vi "UHR-Fleezers Control (host) -TL FB Corrected Ronen semipassive.vi"(0 "Tab Control":T5(tab)=enum."Trap Control (RF)") -> ()   [LabVIEW 2013] (continued)
                    n948 = Wait (ms)(milliseconds to wait=u32 500) -> ()  [unwired: 1 out]
                  }
                  frame #4 {
                    n949 = call "Write to pump.vi"("string"="start", "VISA resource name"=w1515) -> ()  [unwired: 1 out]
                  }
                }
              }
            }
          }
          frame Enabled {
            n950 = call "hamilton_controller.vi"("Open?"=w1517, "valve"=enum16{"A", "B", "C", "D", "ALL"}."A", "action"=T21."MOVE VALVE") -> ()  [unwired: 8 in, 1 out]
          }
        }
      }
      event "Inject Valve B": Value Change {
        n951 = event-data() -> ()  [unwired: 7 out]
        n952 = disable-structure shown="Enabled" {
          disable-tunnel: "Inject Valve B" -> [w1521 w1541]
          frame Disabled {
            n953 = local read "Pump write delay (ms)"() -> (w1523:dbl)
            n954 = flat-sequence {
              tunnel: w1522 -> [w1536]
              tunnel: w1523 -> [w1532]
              tunnel: w1521 -> [_]
              tunnel: w1523 -> [w1538]
              tunnel: w1522 -> [w1539]
              frame #0 {
                n955 = local read "All Pump Parameters"() -> (w1531:T6)
                n956 = Multiply(x=60.0, y="Flush Center Ch Rate (ul/m)") -> (x*y=w1528:dbl)
                n957 = Unbundle By Name(w1531) -> ("Pump 2"=w1537:T33)
                n958 = call "Set pump parameters.vi"("Pump write delay (ms)"=w1532, "Volume (uL)"="Flush Center Ch Volume (uL)", "Rate (uL/h)"=w1528, "Units"=3.0, "Pump #"=2.0, "Pump Parameters In"=w1537, "VISA resource name"=w1536) -> ("Pump Parameters Out"=w1530:T33)  [unwired: 3 in]
                n959 = Bundle By Name(cluster=w1531, "Pump 2"=w1530) -> (w1529:T6)
                n960 = local write "All Pump Parameters"(w1529) -> ()
                n961 = Add(x="Flush Center Ch Volume (uL)", y="Total Volume\nFlushed (uL)") -> (x+y=w1525:dbl)
                n962 = local write "Total Volume\nFlushed (uL)"(w1525) -> ()
              }
              frame #1 {
                n963 = Wait (ms)(milliseconds to wait=w1538) -> ()  [unwired: 1 out]
              }
              frame #2 {
                n964 = call "Write to pump.vi"("string"="start", "VISA resource name"=w1539) -> ()  [unwired: 1 out]
              }
            }
            n965 = local read "Chemyx Syringe Pump Serial Port"() -> (w1522:refnum<visa-resource-name>)
          }
          frame Enabled {
            n966 = call "hamilton_controller.vi"("Open?"=w1541, "valve"=enum16{"A", "B", "C", "D", "ALL"}."B", "action"=T21."MOVE VALVE") -> ()  [unwired: 8 in, 1 out]
          }
        }
      }
      event "Inject Bottom": Value Change {
        n967 = event-data() -> ()  [unwired: 7 out]
        n968 = call "hamilton_controller.vi"("Open?"="Inject Bottom", "valve"=enum16{"A", "B", "C", "D", "ALL"}."C", "action"=T21."MOVE VALVE") -> ()  [unwired: 8 in, 1 out]
      }
      event "Shunt:": Value Change {
        n969 = event-data() -> ()  [unwired: 7 out]
        n970 = call "hamilton_controller.vi"("Open?"="Shunt:", "valve"=enum16{"A", "B", "C", "D", "ALL"}."D", "action"=T21."MOVE VALVE") -> ()  [unwired: 8 in, 1 out]
      }
      event "Flip Green Filter": Value Change {
        n971 = event-data() -> ()  [unwired: 7 out]
        n972 = local write "Flip Green Filter"("Flip Green Filter") -> ()
        n973 = flat-sequence {
          tunnel: w1557 -> [w1562]
          tunnel: w1556 -> [w1561]
          tunnel: [w1559] -> w1554
          tunnel: [w1558] -> w1553
          tunnel: [w1564] -> w1552
          tunnel: w1554 -> [w1564]
          tunnel: [w1563] -> w1551
          tunnel: w1553 -> [w1563]
          tunnel: w1552 -> [w1568]
          tunnel: w1551 -> [w1567]
          tunnel: [w1566] -> w1555
          frame #0 {
            n974 = xnode "Read/Write Control"("FPGA VI Reference In"=w1562, "error in"=w1561, "Green Filter Flipper"=TRUE) -> ("FPGA VI Reference Out"=w1559:T20, "error out"=w1558:errorcluster)
          }
          frame #1 {
            n975 = Wait (ms)(milliseconds to wait=u32 100) -> ()  [unwired: 1 out]
          }
          frame #2 {
            n976 = xnode "Read/Write Control"("FPGA VI Reference In"=w1568, "error in"=w1567, "Green Filter Flipper"=FALSE) -> ("error out"=w1566:errorcluster)  [unwired: 1 out]
          }
        }
      }
      event "Pump 1 contents", "Pump 3 contents": Value Change {
        n977 = event-data() -> ()  [unwired: 7 out]
        n978 = local read "Pump 1 contents"() -> (→"Pump 1 cont disp":string)
        n979 = local read "Pump 3 contents"() -> (→"Pump 3 cont disp":string)
      }
      event "Reset Trap Pos. FB": Value Change {
        n980 = event-data() -> ()  [unwired: 7 out]
        n981 = xnode "Read/Write Control"("FPGA VI Reference In"=w1574, "error in"=w1573, "Trap Pos. FB Reset"="Reset Trap Pos. FB") -> ()  [unwired: 2 out]
      }
      event "Trap Pos. FB ON": Value Change {
        n982 = event-data() -> ()  [unwired: 7 out]
        n983 = xnode "Read/Write Control"("FPGA VI Reference In"=w1589, "error in"=w1588) -> ("FPGA VI Reference Out"=w1586:T20, "BD1 Frequency Out 1"=w1583:u64)  [unwired: 1 out]
        n984 = To Double Precision Float(number=w1583) -> (double precision float=w1582:dbl)
        n985 = Multiply(x=49125000.0, y=6.0) -> (x*y=w1581:dbl)
        n986 = Multiply(x=w1582, y=w1581) -> (x*y=w1579:dbl)
        n987 = Scale By Power Of 2(n=-48, x=w1579) -> (x*2^n=w1578:dbl)
        n988 = Divide(x=w1578, y=1000000.0) -> (x/y=w1575:dbl)
        n989 = flat-sequence {
          tunnel: [w1592] -> w1587
          tunnel: w1586 -> [w1593]
          tunnel: w1583 -> [w1591]
          tunnel: "Trap Pos. FB ON" -> [w1590]
          tunnel: "Trap Pos. FB ON" -> [w1599]
          tunnel: w1587 -> [w1598]
          tunnel: "Trap Pos. FB ON" -> [w1601]
          tunnel: w1575 -> [w1600]
          frame #0 {
            n990 = case shown="False" w1590 {
              tunnel: w1593 -> [w1596 w1597]
              tunnel: [w1595 w1597] -> w1592
              tunnel: w1591 -> [w1594 _]
              frame False {
                n991 = xnode "Read/Write Control"("FPGA VI Reference In"=w1596, "BD 1 Frequency 1"=w1594) -> ("FPGA VI Reference Out"=w1595:T20)  [unwired: 1 in, 1 out]
              }
              frame True {
              }
            }
          }
          frame #1 {
            n992 = xnode "Read/Write Control"("FPGA VI Reference In"=w1598, "Force feedback"=w1599) -> ()  [unwired: 1 in, 2 out]
          }
          frame #2 {
            n993 = case shown="False" w1601 {
              tunnel: w1600 -> [w1603 _]
              frame False {
                n994 = Subtract(x=90.0, y=w1603) -> (x-y=w1602:dbl)
                n995 = property on="Trap Delta (MHz)" class="DigNum (strict)"("Val(Sgnl)"=w1602) -> ()  [unwired: 2 in, 2 out]
              }
              frame True {
              }
            }
          }
        }
      }
      event "Diff. FB.", "Trap Pos. FB Gains", "Trap Pos. FB Mult Factor", "Trap Pos. FB Offset Factor", "Trap Pos FB Negate Action", "Trap Pos FB Monitor\nT1 or T2", "Negate Diff?": Value Change {
        n996 = event-data() -> ()  [unwired: 7 out]
        n997 = xnode "Read/Write Control"("FPGA VI Reference In"=w1615, "error in"=w1614, "Trap Pos. FB Range"="Trap Pos. FB Range", "Trap Pos. FB Gains"="Trap Pos. FB Gains", "Trap Pos. FB Mult Factor"="Trap Pos. FB Mult Factor", "Trap Pos. FB Offset Factor"="Trap Pos. FB Offset Factor", "Trap Pos FB Negate Action"="Trap Pos FB Negate Action", "Trap Pos FB Monitor T1 or T2"="Trap Pos FB Monitor\nT1 or T2", "AI1 X Scale"="Trap Pos. AI1 X Pre-scale", "Negate Diff?"="Negate Diff?", "Diff FB Measurement?"="Diff. FB.") -> ()  [unwired: 2 out]
      }
      event "Trap Pos FB SP": Value Change {
        n998 = event-data() -> ()  [unwired: 7 out]
        n999 = xnode "Read/Write Control"("FPGA VI Reference In"=w1618, "error in"=w1617, "Trap Pos. FB SP"="Trap Pos FB SP") -> ()  [unwired: 2 out]
      }
      event "Set SP to Reading": Value Change {
        n1000 = event-data() -> ()  [unwired: 7 out]
        n1001 = local read "Trap Pos FB Monitor\nT1 or T2"() -> (w1626:bool)
        n1002 = local read "Trap X AI1 (DMA)"() -> (w1629:T13)
        n1003 = local read "Trap X (AI1)"() -> (w1632:T1)
        n1004 = Unbundle By Name(w1632) -> ("Trap 1"=w1631:fxp<+/-,16,1>, "Trap 2"=w1630:fxp<+/-,16,1>)
        n1005 = Unbundle By Name(w1629) -> ("Set 1"=w1628:fxp<+/-,16,1>, "Set 2"=w1627:fxp<+/-,16,1>)
        n1006 = Select(t=w1631, s=w1626, f=w1630) -> (s? t:f=w1625:fxp<+/-,16,1>)
        n1007 = Select(t=w1628, s=w1626, f=w1627) -> (s? t:f=w1624:fxp<+/-,16,1>)
        n1008 = Not(x="Set SP Using...") -> (.not. x?=w1619:bool)
        n1009 = Select(t=w1625, s=w1619, f=w1624) -> (s? t:f=w1620:fxp<+/-,16,1>)
        n1010 = xnode "Read/Write Control"("FPGA VI Reference In"=w1622, "error in"=w1621, "Trap Pos. FB SP"=w1620) -> ()  [unwired: 2 out]
        n1011 = local write "Trap Pos FB SP"(w1620) -> ()
      }
      event "Trap Pos. FB Out Scale 2^n": Value Change {
        n1012 = event-data() -> ()  [unwired: 7 out]
        n1013 = Scale By Power Of 2(n="Trap Pos. FB Out Scale 2^n", x=ext 1.0) -> (x*2^n=w1634:ext)
        n1014 = property on="Trap Pos. FB Mult Factor" class="DigNum (strict)"("Val(Sgnl)"=w1634) -> ()  [unwired: 2 in, 2 out]
      }
      event "Trap Pos FB Int Count": Value Change {
        n1015 = event-data() -> ()  [unwired: 7 out]
        n1016 = xnode "Read/Write Control"("FPGA VI Reference In"=w1639, "error in"=w1638, "Trap Pos FB Int Count"="Trap Pos FB Int Count") -> ()  [unwired: 2 out]
      }
      event "Target Force (pN)", "Setpoint offset\nCorrection values": Value Change {
        n1017 = event-data() -> ()  [unwired: 7 out]
        n1018 = local read "B factor"() -> (w1672:dbl)
        n1019 = To Fixed-Point(number=w1672) -> (fixed-point=w1671:fxp<+/-,16,16>)  [unwired: 1 in]
        n1020 = xnode "Read/Write Control"("FPGA VI Reference In"=w1673, "B factor"=w1671) -> ("BD1 Frequency Out 1"=w1662:u64)  [unwired: 1 in, 2 out]
        n1021 = local read "BD 1 Frequency 2 (MHz)"() -> (w1661:dbl)
        n1022 = local read "Target Force (pN)"() -> (w1647:dbl)
        n1023 = To Double Precision Float(number=w1662) -> (double precision float=w1668:dbl)
        n1024 = Multiply(x=49125000.0, y=6.0) -> (x*y=w1667:dbl)
        n1025 = Multiply(x=w1668, y=w1667) -> (x*y=w1665:dbl)
        n1026 = Scale By Power Of 2(n=-48, x=w1665) -> (x*2^n=w1664:dbl)
        n1027 = Divide(x=w1664, y=1000000.0) -> (x/y=w1660:dbl)
        n1028 = Subtract(x=w1661, y=w1660) -> (x-y=w1659:dbl)
        n1029 = local read "T1 kappa_x (pN/nm)"() -> (w1648:dbl)
        n1030 = local read "T1 alpha_x (nm/V)"() -> (w1649:dbl)
        n1031 = local read "Negate offset difference"() -> (w1650:bool)
        n1032 = local read "Offset file step size"() -> (w1658:dbl)
        n1033 = Multiply(x=w1647, y=2.0) -> (x*y=w1645:dbl)
        n1034 = local read "Setpoint offset\nCorrection values"() -> (w1655:dbl[])
        n1035 = Divide(x=w1659, y=w1658) -> (x/y=w1657:dbl)
        n1036 = Select(t=-1, s=w1650, f=1) -> (s? t:f=w1651:i32)
        n1037 = To Long Integer(number=w1657) -> (32bit integer=w1656:i32)
        n1038 = Multiply(x=w1649, y=w1648) -> (x*y=w1644:dbl)
        n1039 = Divide(x=w1645, y=w1644) -> (x/y=w1643:dbl)
        n1040 = Index Array(array=w1655, index=w1656) -> (element=w1654:dbl)
        n1041 = Multiply(x=w1651, y=w1654) -> (x*y=w1642:dbl)
        n1042 = Add(x=w1643, y=w1642) -> (x+y=w1641:dbl)
        n1043 = To Fixed-Point(number=w1641) -> (fixed-point=w1640:fxp<+/-,16,1>)  [unwired: 1 in]
        n1044 = property on="Trap Pos FB SP" class="DigNum (strict)"("Val(Sgnl)"=w1640) -> ()  [unwired: 2 in, 2 out]
      }
      event "Read setpoint correction\nfile": Value Change {
        n1045 = event-data() -> ()  [unwired: 7 out]
        n1046 = local write "Read setpoint correction\nfile"(FALSE) -> ()
        n1047 = Open/Create/Replace File(file path (use dialog)="Setpoint correction\noffset file", operation (0:open)=T24."open", access (0:read/write)=enum16{"read/write", "read-only", "write-only"}."read-only") -> (refnum out=w1698:refnum<file>)  [unwired: 1 in, 4 out]
        n1048 = Deny Access(7:w1698) -> (3:w1696:refnum<file>)  [unwired: 1 in, 2 out]
        n1049 = Read from Binary File(5:0.0, 9:T30."big-endian, network order" ("byte order (0:big-endian, network order)"), 10:-1 ("count (1)"), 11:w1696) -> (2:w1689:dbl[], 3:w1695:refnum<file>)  [unwired: 1 in, 3 out]
        n1050 = Close File(refnum=w1695) -> ()  [unwired: 1 in, 2 out]
        n1051 = Index Array(array=w1689, index=0) -> (element=w1685:dbl)
        n1052 = local write "Offset file step size"(w1685) -> ()
        n1053 = Array Subset(array=w1689, index=3) -> (w1688:dbl[])  [unwired: 1 in]
        n1054 = local read "T1 kappa_x (pN/nm)"() -> (w1683:dbl)
        n1055 = local read "T1 alpha_x (nm/V)"() -> (w1684:dbl)
        n1056 = local read "T2 alpha_x (nm/V)"() -> (w1682:dbl)
        n1057 = local read "T2 kappa_x (pN/nm)"() -> (w1681:dbl)
        n1058 = Decimate 1D Array(w1688) -> (w1676:dbl[], w1677:dbl[])  [unwired: 1 out]
        n1059 = local read "Offset Values"() -> (w1687:T14)
        n1060 = Multiply(x=w1684, y=w1683) -> (x*y=w1679:dbl)
        n1061 = Multiply(x=w1682, y=w1681) -> (x*y=w1680:dbl)
        n1062 = Bundle By Name(cluster=w1687, "Trap 1X offset"=w1676, "Trap 2X offset"=w1677) -> (w1686:T14)
        n1063 = Divide(x=w1680, y=w1679) -> (x/y=w1678:dbl)
        n1064 = property on="B factor" class="DigNum (strict)"("Val(Sgnl)"=w1678) -> ()  [unwired: 2 in, 2 out]
        n1065 = Multiply(x=w1677, y=w1678) -> (x*y=w1675:dbl[])
        n1066 = local write "Offset Values"(w1686) -> ()
        n1067 = Subtract(x=w1676, y=w1675) -> (x-y=w1674:dbl[])
        n1068 = property on="Setpoint offset\nCorrection values" class="Arr (strict)"("Val(Sgnl)"=w1674) -> ()  [unwired: 2 in, 2 out]
      }
      event "MCL Tracking": Value Change {
        n1069 = event-data() -> ()  [unwired: 7 out]
        n1070 = case shown="True" "MCL Tracking" {
          frame False {
            n1071 = local read "Current MCL (V)"() -> (w1703:dbl)
            n1072 = local write "AO2"(w1703) -> ()
          }
          frame True {
            n1073 = local read "BD 1 Frequency 1 (MHz)"() -> (→"Zero T1 position":dbl)
            n1074 = local read "AO2"() -> (→"Zero MCL x position":dbl)
          }
        }
      }
    }
    "error out 2" <- w754
    n1075 = node-c288() -> ()  [unwired: 1 in, 1 out]
  }
  n1076 = timed-loop "Run Scripts, including: stage motion" {
    timing: w89 -> [_]
    timing-out: [_] -> w88
    tunnel: w44 -> [_]
    stop <- w1707 stop-if-true
    n1077 = node-c288() -> ()  [unwired: 1 in, 1 out]
    n1078 = event shown="[2] \"Cal/Data Acq. Spot\": Value Change" {
      selector: _ -> [_ _ _ _ _ _ _ _ _ _ _ _]
      dyn-events: _ -> [_ _ _ _ _ _ _ _ _ _ _ _]
      timeout: 50 -> [_ _ _ _ _ _ _ _ _ _ _ _]
      tunnel: ["Move Cap. 1 (DNA Top)" _ "Cal/Data Acq. Spot" "Dump Beads" "Dip for Protein" _ "Got ADig bead" "Got DNA bead" "Take Stepping Data" _ "Take Detection Laser\nImage" _] -> _
      tunnel: [_ _ _ _ _ _ _ _ _ _ _ w1915] -> w1707
      event "Move Cap. 1 (DNA Top)": Value Change {
        n1079 = event-data() -> ()  [unwired: 1 in, 5 out]
        n1080 = local write "Move Cap. 1 (DNA Top)"(FALSE ("Move Cap. 1 (DNA Right)")) -> ()
        n1081 = flat-sequence {
          tunnel: "Cap 1 Samp Flow ON" -> [w1713]
          frame #0 {
            n1082 = local write "Stage Moving"(FALSE ("Stage Moving")) -> ()
            n1083 = case "stop flow" shown="True" w1713 {
              frame False {
              }
              frame True {
                n1084 = call "hamilton_controller.vi"("Open?"=FALSE, "valve"=enum16{"A", "B", "C", "D", "ALL"}."C", "action"=T21."MOVE VALVE") -> ()  [unwired: 8 in, 1 out]
              }
            }
            n1085 = case shown="True" TRUE {
              tunnel: "Cap 1 T ON" -> [w1722 w1723]
              frame False {
                n1086 = property on="Trap 1 (ON/OFF)" class="Bool (strict)"("Val(Sgnl)"=w1722) -> ()  [unwired: 2 in, 2 out]
              }
              frame True {
                n1087 = property on="Trap 2 (ON/OFF)" class="Bool (strict)"("Val(Sgnl)"=w1723) -> ()  [unwired: 2 in, 2 out]
              }
            }
            n1088 = call <vilib>:"Beep.vi"() -> ()  [unwired: 3 in, 9 out]
            n1089 = case shown="True" "Cap 1 Flow ON" {
              frame False {
              }
              frame True {
                n1090 = property on="Main:" class="Bool (strict)"("Val(Sgnl)"=TRUE ("Value (Signaling)")) -> ()  [unwired: 2 in, 2 out]
              }
            }
          }
        }
      }
      event Timeout {
        n1091 = event-data() -> ()  [unwired: 1 in, 2 out]
      }
      event "Cal/Data Acq. Spot": Value Change {
        # "wait for calibration file\nto be written"
        # "signal save cal true\nthis tells the data \nacquisition loop to\nstart sending the data\nto a calibration file"
        # "separate traps to\nthe desired trap delta"
        # "move stage to data acquisition spot"
        # "CHANGE FISH FOR TETHER BACK\nTO TRUE VALUE HERE."
        n1092 = event-data() -> ()  [unwired: 1 in, 5 out]
        n1093 = local write "Cal/Data Acq. Spot"(FALSE ("Cal/Data Acq. Spot")) -> ()
        n1094 = flat-sequence {
          tunnel: ["Cal @ (MHz)"] -> w1724
          tunnel: w1724 -> [w1734]
          tunnel: w1724 -> [w1755]
          frame #0 {
            n1095 = property on="Trap Delta (MHz)" class="DigNum (strict)"("Val(Sgnl)"="Cal @ (MHz)") -> ()  [unwired: 2 in, 2 out]
            n1096 = call <vilib>:"Beep.vi"() -> ()  [unwired: 3 in, 9 out]
          }
          frame #1 {
            n1097 = Wait (ms)(milliseconds to wait=u32 100) -> ()  [unwired: 1 out]
          }
          frame #2 {
            n1098 = property on="Save Calibration" class="Bool (strict)"("Val(Sgnl)"=TRUE ("Value (Signaling)")) -> ()  [unwired: 2 in, 2 out]
          }
          frame #3 {
            n1099 = Wait (ms)(milliseconds to wait=u32 4000) -> ()  [unwired: 1 out]
          }
          frame #4 {
            n1100 = while {
              stop <- w1731 stop-if-true
              n1101 = local read "Saving..."() -> (w1732:bool)
              n1102 = Wait (ms)(milliseconds to wait=u32 100) -> ()  [unwired: 1 out]
              n1103 = Not(x=w1732) -> (.not. x?=w1731:bool)
            }
          }
          frame #5 {
            n1104 = case shown="True" "W/ Offset 1" {
              tunnel: w1734 -> [_ w1736]
              frame False {
              }
              frame True {
                n1105 = stacked-sequence {
                  tunnel: w1736 -> [_ _ _ _ _ _ _ w1753]
                  frame #0 {
                    n1106 = Replace Array Subset(array=u32[] [0] ("Index Values"), new element="Offset 1 Set", index=0) -> (w1737:u32[])
                    n1107 = property on="Saved AOD Raster Scan Parameter Sets" class="Arr (strict)"("Index Values"=w1737) -> ()  [unwired: 2 in, 2 out]
                    n1108 = property on="Trap Delta (MHz)" class="DigNum (strict)"("Val(Sgnl)"="Offset 1 Start (MHz)") -> ()  [unwired: 2 in, 2 out]
                  }
                  frame #1 {
                    n1109 = Wait (ms)(milliseconds to wait=u32 200) -> ()  [unwired: 1 out]
                  }
                  frame #2 {
                    n1110 = property on="Load parameters" class="Bool (strict)"("Val(Sgnl)"=TRUE ("Value (Signaling)")) -> ()  [unwired: 2 in, 2 out]
                  }
                  frame #3 {
                    n1111 = Wait (ms)(milliseconds to wait=u32 200) -> ()  [unwired: 1 out]
                  }
                  frame #4 {
                    n1112 = property on="Trap Raster Scan" class="Bool (strict)"("Val(Sgnl)"=TRUE ("Value (Signaling)")) -> ()  [unwired: 2 in, 2 out]
                  }
                  frame #5 {
                    n1113 = Wait (ms)(milliseconds to wait=u32 2000) -> ()  [unwired: 1 out]
                  }
                  frame #6 {
                    n1114 = while {
                      stop <- w1750 stop-if-true
                      n1115 = local read "Raster Scanning..."() -> (w1752:bool)
                      n1116 = local read "Saving..."() -> (w1748:bool)
                      n1117 = Wait (ms)(milliseconds to wait=u32 100) -> ()  [unwired: 1 out]
                      n1118 = Not(x=w1748) -> (.not. x?=w1747:bool)
                      n1119 = Not(x=w1752) -> (.not. x?=w1749:bool)
                      n1120 = And(x=w1749, y=w1747) -> (x .and. y?=w1750:bool)
                    }
                  }
                  frame #7 {
                    n1121 = property on="Trap Delta (MHz)" class="DigNum (strict)"("Val(Sgnl)"=w1753) -> ()  [unwired: 2 in, 2 out]
                  }
                }
              }
            }
          }
          frame #6 {
            n1122 = local read "Save ave N"() -> (w1754:dbl)
            n1123 = case shown="True" "W/ Offset 2" {
              tunnel: w1755 -> [_ w1761]
              tunnel: w1754 -> [_ w1760]
              frame False {
                n1124 = Multiply(x="Cal read wait (s)", y=u32 1000 ("milliseconds to wait")) -> (x*y=w1758:u32)
                n1125 = Wait (ms)(milliseconds to wait=w1758) -> ()  [unwired: 1 out]
              }
              frame True {
                n1126 = stacked-sequence {
                  tunnel: w1761 -> [_ _ _ _ _ _ _ _ _ w1782 _ _]
                  tunnel: w1760 -> [_ _ _ _ _ _ _ _ _ w1780 _ _]
                  frame #0 {
                    n1127 = property on="Save ave N" class="DigNum (strict)"("Val(Sgnl)"=1.0 ("Value (Signaling)")) -> ()  [unwired: 2 in, 2 out]
                  }
                  frame #1 {
                    n1128 = Wait (ms)(milliseconds to wait=u32 500) -> ()  [unwired: 1 out]
                  }
                  frame #2 {
                    n1129 = property on="Trap Delta (MHz)" class="DigNum (strict)"("Val(Sgnl)"="Offset 2 Start (MHz)") -> ()  [unwired: 2 in, 2 out]
                    n1130 = Replace Array Subset(array=u32[] [0] ("Index Values"), new element="Offset 2 Set", index=0) -> (w1766:u32[])
                    n1131 = property on="Saved AOD Raster Scan Parameter Sets" class="Arr (strict)"("Index Values"=w1766) -> ()  [unwired: 2 in, 2 out]
                  }
                  frame #3 {
                    n1132 = Wait (ms)(milliseconds to wait=u32 500) -> ()  [unwired: 1 out]
                  }
                  frame #4 {
                    n1133 = property on="Load parameters" class="Bool (strict)"("Val(Sgnl)"=TRUE ("Value (Signaling)")) -> ()  [unwired: 2 in, 2 out]
                  }
                  frame #5 {
                    n1134 = Wait (ms)(milliseconds to wait=u32 500) -> ()  [unwired: 1 out]
                  }
                  frame #6 {
                    n1135 = property on="Trap Raster Scan" class="Bool (strict)"("Val(Sgnl)"=TRUE ("Value (Signaling)")) -> ()  [unwired: 2 in, 2 out]
                  }
                  frame #7 {
                    n1136 = Wait (ms)(milliseconds to wait=u32 2000) -> ()  [unwired: 1 out]
                  }
                  frame #8 {
                    n1137 = while {
                      stop <- w1775 stop-if-true
                      n1138 = local read "Raster Scanning..."() -> (w1778:bool)
                      n1139 = local read "Saving..."() -> (w1776:bool)
                      n1140 = Wait (ms)(milliseconds to wait=u32 100) -> ()  [unwired: 1 out]
                      n1141 = Not(x=w1776) -> (.not. x?=w1774:bool)
                      n1142 = Not(x=w1778) -> (.not. x?=w1777:bool)
                      n1143 = And(x=w1777, y=w1774) -> (x .and. y?=w1775:bool)
                    }
                  }
                  frame #9 {
                    n1144 = property on="Trap Delta (MHz)" class="DigNum (strict)"("Val(Sgnl)"=w1782) -> ()  [unwired: 2 in, 2 out]
                    n1145 = property on="Saved AOD Raster Scan Parameter Sets" class="Arr (strict)"("Index Values"=u32[] [0]) -> ()  [unwired: 2 in, 2 out]
                    n1146 = property on="Save ave N" class="DigNum (strict)"("Val(Sgnl)"=w1780) -> ()  [unwired: 2 in, 2 out]
                  }
                  frame #10 {
                    n1147 = Wait (ms)(milliseconds to wait=u32 500) -> ()  [unwired: 1 out]
                  }
                  frame #11 {
                    n1148 = property on="Load parameters" class="Bool (strict)"("Val(Sgnl)"=TRUE ("Value (Signaling)")) -> ()  [unwired: 2 in, 2 out]
                  }
                }
              }
            }
          }
          frame #7 {
            n1149 = property on="Read Cal" class="Bool (strict)"("Val(Sgnl)"=TRUE ("Value (Signaling)")) -> ()  [unwired: 2 in, 2 out]
          }
          frame #8 {
            n1150 = Wait (ms)(milliseconds to wait=u32 500) -> ()  [unwired: 1 out]
          }
          frame #9 {
            n1151 = property on="Fish for Tether" class="Bool (strict)"("Val(Sgnl)"=FALSE ("Value (Signaling)")) -> ()  [unwired: 2 in, 2 out]
          }
        }
      }
      event "Dump Beads": Value Change {
        # "SCRIPT TO REMOVE BOTH BEADS FROM THE TRAPS. TURNS ON LIGHT WHICH INDICATES THAT STAGE IS MOVING. THEN STOPS SAVING DATA. \nSETS Sample Channel Flow TO TRUE. STOPS INTERLACING GREEN FLUORESCENCE. TURNS OFF Tether INDICATOR BECAUSE WE ARE THROWING IT\nAWAY. SHUTS OFF TRAP POSITION FEEDBACK."
        n1152 = event-data() -> ()  [unwired: 1 in, 5 out]
        n1153 = flat-sequence {
          frame #0 {
            w1789 = FALSE ("Fl. Triggered...")
            w1790 = TRUE ("Stage Moving")
            n1154 = local read "Saving..."() -> (w1791:bool)
            n1155 = local write "Fl. Triggered..."(w1789) -> ()
            n1156 = local write "Stage Moving"(w1790) -> ()
            n1157 = local write "Tether"(w1789) -> ()
            n1158 = property on="Green Laser ON/Interlacing" class="Bool (strict)"("Val(Sgnl)"=w1789) -> ()  [unwired: 2 in, 2 out]
            n1159 = property on="Trap Pos. FB ON" class="Bool (strict)"("Val(Sgnl)"=w1789) -> ()  [unwired: 2 in, 2 out]
            n1160 = property on="Inject Bottom" class="Bool (strict)"("Val(Sgnl)"=w1790) -> ()  [unwired: 2 in, 2 out]
            n1161 = local write "Stop Saving"(w1791) -> ()
          }
          frame #1 {
            w1792 = FALSE ("Value (Signaling)")
            # "TURNS TRAPS OFF SO THAT\nBEADS REMAIN AT DUMP \nBEADS POSITION"
            n1162 = property on="Trap 1 (ON/OFF)" class="Bool (strict)"("Val(Sgnl)"=w1792) -> ()  [unwired: 2 in, 2 out]
            n1163 = property on="Trap 2 (ON/OFF)" class="Bool (strict)"("Val(Sgnl)"=w1792) -> ()  [unwired: 2 in, 2 out]
            n1164 = call <vilib>:"Beep.vi"() -> ()  [unwired: 3 in, 9 out]
          }
          frame #2 {
            n1165 = property on="Goto Bottom (F7)" class="Bool (strict)"("Val(Sgnl)"=TRUE ("Value (Signaling)")) -> ()  [unwired: 2 in, 2 out]
          }
          frame #3 {
            n1166 = Wait (ms)(milliseconds to wait=u32 8000) -> ()  [unwired: 1 out]
          }
          frame #4 {
            n1167 = property on="Trap Delta (MHz)" class="DigNum (strict)"("Val(Sgnl)"=20.0 ("Value (Signaling)")) -> ()  [unwired: 2 in, 2 out]
          }
          frame #5 {
            n1168 = property on="Trap 2 (ON/OFF)" class="Bool (strict)"("Val(Sgnl)"=TRUE ("Value (Signaling)")) -> ()  [unwired: 2 in, 2 out]
          }
          frame #6 {
            n1169 = property on="Inject Bottom" class="Bool (strict)"("Val(Sgnl)"=FALSE ("Value (Signaling)")) -> ()  [unwired: 2 in, 2 out]
          }
        }
      }
      event "Dip for Protein": Value Change {
        n1170 = event-data() -> ()  [unwired: 1 in, 5 out]
        n1171 = flat-sequence {
          frame #0 {
            n1172 = case shown="True" "Move Trap Before?" {
              frame False {
              }
              frame True {
                n1173 = property on="Trap Delta (MHz)" class="DigNum (strict)"("Val(Sgnl)"="Dip Trap Delta 1 (MHz)") -> ()  [unwired: 2 in, 2 out]
              }
            }
          }
          frame #1 {
            n1174 = Multiply(x="Duration (s)", y=1000.0) -> (x*y=w1801:dbl)
            n1175 = Wait (ms)(milliseconds to wait=w1801) -> ()  [unwired: 1 out]
          }
          frame #2 {
            n1176 = case shown="True" "Move Trap After?" {
              frame False {
              }
              frame True {
                n1177 = property on="Trap Delta (MHz)" class="DigNum (strict)"("Val(Sgnl)"="Dip Trap Delta 2 (MHz)") -> ()  [unwired: 2 in, 2 out]
              }
            }
          }
          frame #3 {
            n1178 = case shown="True" "Green ON After?" {
              frame False {
              }
              frame True {
                n1179 = property on="Green Laser ON/Interlacing" class="Bool (strict)"("Val(Sgnl)"=TRUE ("Value (Signaling)")) -> ()  [unwired: 2 in, 2 out]
              }
            }
          }
          frame #4 {
            n1180 = Wait (ms)(milliseconds to wait=u32 500) -> ()  [unwired: 1 out]
          }
          frame #5 {
            n1181 = case shown="True" "Save Data After?" {
              frame False {
              }
              frame True {
                n1182 = property on="Start Saving" class="Bool (strict)"("Val(Sgnl)"=TRUE ("Value (Signaling)")) -> ()  [unwired: 2 in, 2 out]
              }
            }
          }
        }
      }
      event "Profile": Value Change {
        n1183 = event-data() -> ()  [unwired: 1 in, 5 out]
        n1184 = flat-sequence {
          frame #0 {
            w1811 = 0.0 ("element")
            n1185 = Build Array(w1811, "Y change (mm)", w1811) -> ()  [unwired: 1 out]
          }
          frame #1 {
            # "stop saving"
            n1186 = local write "Stop Saving"(TRUE ("Stop Saving")) -> ()
            n1187 = local write "Stage Moving"(FALSE ("Stage Moving")) -> ()
          }
        }
      }
      event "Got ADig bead": Value Change {
        n1188 = event-data() -> ()  [unwired: 1 in, 5 out]
        n1189 = property on="Move Cap. 1 (DNA Top)" class="Bool (strict)"("Val(Sgnl)"=TRUE ("Value (Signaling)")) -> ()  [unwired: 2 in, 2 out]
        n1190 = property on="Inject Top:" class="Bool (strict)"("Val(Sgnl)"=FALSE ("Value (Signaling)")) -> ()  [unwired: 2 in, 2 out]
      }
      event "Got DNA bead": Value Change {
        n1191 = event-data() -> ()  [unwired: 1 in, 5 out]
        n1192 = property on="Cal/Data Acq. Spot" class="Bool (strict)"("Val(Sgnl)"=TRUE ("Value (Signaling)")) -> ()  [unwired: 2 in, 2 out]
        n1193 = property on="Main:" class="Bool (strict)"("Val(Sgnl)"=FALSE ("Value (Signaling)")) -> ()  [unwired: 2 in, 2 out]
      }
      event "Take Stepping Data": Value Change {
        n1194 = event-data() -> ()  [unwired: 1 in, 5 out]
        n1195 = local read "Save ave N"() -> (w1829:dbl)
        n1196 = flat-sequence {
          tunnel: w1829 -> [w1831]
          tunnel: [w1831] -> w1824
          tunnel: [w1833] -> w1825
          tunnel: w1824 -> [w1833]
          tunnel: [w1835] -> w1826
          tunnel: w1825 -> [w1835]
          tunnel: [w1838] -> w1827
          tunnel: w1826 -> [w1838]
          tunnel: [w1840] -> w1828
          tunnel: w1827 -> [w1840]
          tunnel: [w1842] -> w1822
          tunnel: w1828 -> [w1842]
          tunnel: w1822 -> [w1845]
          tunnel: [w1845] -> w1821
          tunnel: w1821 -> [w1846]
          tunnel: [w1846] -> w1823
          tunnel: w1823 -> [w1852]
          frame #0 {
            n1197 = property on="Save ave N" class="DigNum (strict)"("Val(Sgnl)"="Save ave factor") -> ()  [unwired: 2 in, 2 out]
          }
          frame #1 {
            n1198 = Wait (ms)(milliseconds to wait=u32 100) -> ()  [unwired: 1 out]
          }
          frame #2 {
            n1199 = local read "Offset 2 Start (MHz)"() -> (w1837:dbl)
            n1200 = property on="Saved AOD Raster Scan Parameter Sets" class="Arr (strict)"("Index Values"=u32[] [2]) -> ()  [unwired: 2 in, 2 out]
            n1201 = property on="Trap Delta (MHz)" class="DigNum (strict)"("Val(Sgnl)"=w1837) -> ()  [unwired: 2 in, 2 out]
          }
          frame #3 {
            n1202 = property on="Load parameters" class="Bool (strict)"("Val(Sgnl)"=TRUE ("Value (Signaling)")) -> ()  [unwired: 2 in, 2 out]
          }
          frame #4 {
            n1203 = Wait (ms)(milliseconds to wait=u32 100) -> ()  [unwired: 1 out]
          }
          frame #5 {
            n1204 = property on="Trap Raster Scan" class="Bool (strict)"("Val(Sgnl)"=TRUE ("Value (Signaling)")) -> ()  [unwired: 2 in, 2 out]
          }
          frame #6 {
            n1205 = Wait (ms)(milliseconds to wait=u32 1000) -> ()  [unwired: 1 out]
          }
          frame #7 {
            n1206 = while {
              stop <- w1849 stop-if-true
              n1207 = local read "Raster Scanning..."() -> (w1851:bool)
              n1208 = local read "Saving..."() -> (w1850:bool)
              n1209 = Not(x=w1850) -> (.not. x?=w1847:bool)
              n1210 = Not(x=w1851) -> (.not. x?=w1848:bool)
              n1211 = And(x=w1848, y=w1847) -> (x .and. y?=w1849:bool)
            }
          }
          frame #8 {
            n1212 = property on="Save ave N" class="DigNum (strict)"("Val(Sgnl)"=w1852) -> ()  [unwired: 2 in, 2 out]
          }
        }
      }
      event "Step Size (nm)": Value Change {
        n1213 = event-data() -> ()  [unwired: 1 in, 5 out]
        n1214 = flat-sequence {
          frame #0 {
            n1215 = property on="Saved AOD Raster Scan Parameter Sets" class="Arr (strict)"("Index Values"=u32[] [1]) -> ()  [unwired: 2 in, 2 out]
          }
          frame #1 {
            n1216 = Multiply(x="N Steps", y="Step Size (nm)") -> (x*y=w1854:dbl)
            n1217 = property on="Scan Speed AOD (nm/s) 2" class="DigNum (strict)"("Value"="Step Size (nm)") -> ()  [unwired: 2 in, 2 out]
            n1218 = property on="Step Size AOD (nm) 2" class="DigNum (strict)"("Value"="Step Size (nm)") -> ()  [unwired: 2 in, 2 out]
            n1219 = property on="Scan Range AOD (nm) 2" class="DigNum (strict)"("Value"=w1854) -> ()  [unwired: 2 in, 2 out]
          }
        }
      }
      event "Take Detection Laser\nImage": Value Change {
        n1220 = event-data() -> ()  [unwired: 1 in, 5 out]
        n1221 = flat-sequence {
          tunnel: [w1882] -> w1872
          tunnel: [w1881] -> w1865
          tunnel: [w1880] -> w1857
          tunnel: [w1885] -> w1873
          tunnel: w1872 -> [w1885]
          tunnel: [w1884] -> w1866
          tunnel: w1865 -> [w1884]
          tunnel: [w1883] -> w1858
          tunnel: w1857 -> [w1883]
          tunnel: [w1889] -> w1874
          tunnel: w1873 -> [w1889]
          tunnel: [w1888] -> w1867
          tunnel: w1866 -> [w1888]
          tunnel: [w1887] -> w1859
          tunnel: w1858 -> [w1887]
          tunnel: [w1895] -> w1875
          tunnel: w1874 -> [w1895]
          tunnel: [w1894] -> w1868
          tunnel: w1867 -> [w1894]
          tunnel: [w1893] -> w1860
          tunnel: w1859 -> [w1893]
          tunnel: [w1899] -> w1876
          tunnel: w1875 -> [w1899]
          tunnel: [w1898] -> w1869
          tunnel: w1868 -> [w1898]
          tunnel: [w1897] -> w1861
          tunnel: w1860 -> [w1897]
          tunnel: [w1903] -> w1877
          tunnel: w1876 -> [w1903]
          tunnel: [w1902] -> w1870
          tunnel: w1869 -> [w1902]
          tunnel: [w1901] -> w1862
          tunnel: w1861 -> [w1901]
          tunnel: [w1907] -> w1878
          tunnel: w1877 -> [w1907]
          tunnel: [w1906] -> w1871
          tunnel: w1870 -> [w1906]
          tunnel: [w1905] -> w1863
          tunnel: w1862 -> [w1905]
          tunnel: w1878 -> [w1913]
          tunnel: w1871 -> [w1912]
          tunnel: [w1910] -> w1864
          tunnel: w1863 -> [w1910]
          tunnel: w1864 -> [w1914]
          frame #0 {
            n1222 = local read "Green Laser ON/Interlacing"() -> (w1882:bool)
            n1223 = local read "Green laser mode"() -> (w1881:enum32{"Laser ON", "Laser OFF", "Interlace"})
            n1224 = local read "Green FB On/Off"() -> (w1880:bool)
          }
          frame #1 {
            n1225 = property on="Green FB On/Off" class="Bool (strict)"("Val(Sgnl)"=FALSE ("Value (Signaling)")) -> ()  [unwired: 2 in, 2 out]
          }
          frame #2 {
            n1226 = property on="Green Laser ON/Interlacing" class="Bool (strict)"("Val(Sgnl)"=TRUE ("Value (Signaling)")) -> ()  [unwired: 2 in, 2 out]
            n1227 = property on="Flip Green Filter" class="Bool (strict)"("Val(Sgnl)"=TRUE ("Value (Signaling)")) -> ()  [unwired: 2 in, 2 out]
            n1228 = property on="Green laser mode" class="RadioBtnsControl (strict)"("Val(Sgnl)"=enum32{"Laser ON", "Laser OFF", "Interlace"}."Laser ON" ("Value (Signaling)")) -> ()  [unwired: 2 in, 2 out]
          }
          frame #3 {
            n1229 = Wait (ms)(milliseconds to wait=u32 500) -> ()  [unwired: 1 out]
          }
          frame #4 {
            n1230 = property on="Confocal Image" class="Bool (strict)"("Val(Sgnl)"=TRUE ("Value (Signaling)")) -> ()  [unwired: 2 in, 2 out]
          }
          frame #5 {
            n1231 = Wait (ms)(milliseconds to wait=u32 2000) -> ()  [unwired: 1 out]
          }
          frame #6 {
            n1232 = while {
              stop <- w1908 stop-if-true
              n1233 = local read "Saving..."() -> (w1909:bool)
              n1234 = Not(x=w1909) -> (.not. x?=w1908:bool)
            }
          }
          frame #7 {
            n1235 = property on="Flip Green Filter" class="Bool (strict)"("Val(Sgnl)"=TRUE ("Value (Signaling)")) -> ()  [unwired: 2 in, 2 out]
            n1236 = property on="Green Laser ON/Interlacing" class="Bool (strict)"("Val(Sgnl)"=w1913) -> ()  [unwired: 2 in, 2 out]
            n1237 = property on="Green laser mode" class="RadioBtnsControl (strict)"("Val(Sgnl)"=w1912) -> ()  [unwired: 2 in, 2 out]
          }
          frame #8 {
            n1238 = property on="Green FB On/Off" class="Bool (strict)"("Val(Sgnl)"=w1914) -> ()  [unwired: 2 in, 2 out]
          }
        }
      }
      event "Stop All": Value Change {
        n1239 = event-data() -> ()  [unwired: 1 in, 5 out]
        n1240 = local read "Stop All"() -> (w1915:bool)
      }
    }
    n1241 = node-c288() -> ()  [unwired: 1 in, 1 out]
  }
  n1242 = node-c288() -> (w96:T25)  [unwired: 4 out]
  n1243 = timed-loop "Mouse control: trap position (AOM deflection), set confocal spot from image" {
    tunnel: [w1917] -> w54
    tunnel: w44 -> [w1916]
    timing: w96 -> [_]
    timing-out: [_] -> w95
    stop <- w1917 stop-if-true
    n1244 = node-c288() -> ()  [unwired: 2 out]
    n1245 = event shown="[0] \"Pane\": Mouse Down" {
      selector: _ -> [_ _]
      dyn-events: _ -> [_ _]
      timeout: _ -> [_ _]
      tunnel: w1916 -> [w1920 _]
      event Mouse Down {
        n1246 = event-data() -> ("Time"=w1922:u32, "Coords"=w1921:T8, "Button"=w1923:u16)  [unwired: 6 out]
        n1247 = case shown="1" w1923 {
          tunnel: w1922 -> [_ _ w2026]
          tunnel: w1921 -> [_ w1960 w2024]
          tunnel: w1920 -> [_ _ w2022]
          frame 0, Default {
          }
          frame 1 {
            n1248 = property on="APD 2" class="ImageControl"() -> ("Displayed Image Position"=w1930:cluster{"Left":i32, "Top":i32})  [unwired: 2 in, 2 out]
            n1249 = property on="APD 1" class="ImageControl"() -> ("Displayed Image Position"=w1959:cluster{"Left":i32, "Top":i32})  [unwired: 2 in, 2 out]
            n1250 = property on="Detection Laser X" class="ImageControl"() -> ("Displayed Image Position"=w1956:cluster{"Left":i32, "Top":i32})  [unwired: 2 in, 2 out]
            n1251 = property on="Detection Laser Y" class="ImageControl"() -> ("Displayed Image Position"=w1955:cluster{"Left":i32, "Top":i32})  [unwired: 2 in, 2 out]
            n1252 = property on="APD 2" class="ImageControl"() -> ("Displayed Image Size"=w1929:cluster{"Width":u32, "Height":u32})  [unwired: 2 in, 2 out]
            n1253 = property on="APD 1" class="ImageControl"() -> ("Displayed Image Size"=w1957:cluster{"Width":u32, "Height":u32})  [unwired: 2 in, 2 out]
            n1254 = property on="Detection Laser X" class="ImageControl"() -> ("Displayed Image Size"=w1958:cluster{"Width":u32, "Height":u32})  [unwired: 2 in, 2 out]
            n1255 = property on="Detection Laser Y" class="ImageControl"() -> ("Displayed Image Size"=w1954:cluster{"Width":u32, "Height":u32})  [unwired: 2 in, 2 out]
            n1256 = Unbundle By Name(w1929) -> ("Width"=w1926:u32, "Height"=w1925:u32)
            n1257 = Unbundle By Name(w1930) -> ("Left"=w1928:i32, "Top"=w1927:i32)
            n1258 = Unbundle By Name(w1957) -> ("Width"=w1951:u32, "Height"=w1950:u32)
            n1259 = Unbundle By Name(w1958) -> ("Width"=w1947:u32, "Height"=w1946:u32)
            n1260 = Unbundle By Name(w1954) -> ("Width"=w1943:u32, "Height"=w1942:u32)
            n1261 = Unbundle By Name(w1959) -> ("Left"=w1953:i32, "Top"=w1952:i32)
            n1262 = Unbundle By Name(w1956) -> ("Left"=w1949:i32, "Top"=w1948:i32)
            n1263 = Unbundle By Name(w1955) -> ("Left"=w1945:i32, "Top"=w1944:i32)
            n1264 = Bundle("Left"=w1928, "Top"=w1927, "Width"=w1926, "Height"=w1925) -> (w1924:T34)  [unwired: 1 in]
            n1265 = Bundle("Left"=w1953, "Top"=w1952, "Width"=w1951, "Height"=w1950) -> (w1941:T34)  [unwired: 1 in]
            n1266 = Bundle("Left"=w1949, "Top"=w1948, "Width"=w1947, "Height"=w1946) -> (w1940:T34)  [unwired: 1 in]
            n1267 = Bundle("Left"=w1945, "Top"=w1944, "Width"=w1943, "Height"=w1942) -> (w1939:T34)  [unwired: 1 in]
            n1268 = Build Cluster Array(w1924, w1941, w1940, w1939) -> (w1938:T35)
            n1269 = for {
              tunnel: w1960 -> [w1971]
              tunnel: w1938 -> [w1972] mode=indexing
              shift-right: [w1969] -> w1936
              shift-left: TRUE -> [w1970]
              shift-right: [w1968] -> w1934
              shift-left: _ -> [w1964]
              shift-right: [w1967] -> w1933
              shift-left: _ -> [w1963]
              shift-right: [w1966] -> w1932
              shift-left: _ -> [w1962]
              shift-right: [w1965] -> w1931
              shift-left: _ -> [w1961]
              n1270 = case shown="True" w1970 {
                selector: w1970 -> [w1977 _]
                tunnel: w1972 -> [_ w1986]
                tunnel: w1971 -> [_ w1984]
                tunnel: [w1977 w1982] -> w1969
                tunnel: [w1976 w1981] -> w1968
                tunnel: [w1975 w1980] -> w1967
                tunnel: [w1974 w1979] -> w1966
                tunnel: [w1973 w1978] -> w1965
                tunnel: w1964 -> [w1976 _]
                tunnel: w1963 -> [w1975 _]
                tunnel: w1962 -> [w1974 _]
                tunnel: w1961 -> [w1973 _]
                frame False {
                }
                frame True {
                  n1271 = Unbundle(w1986) -> (w1985:T34)
                  n1272 = call "isclickinwindow.vi"("Image Param"=w1985, "Point32"=w1984) -> ("4 Y"=w1978:i32, "3 Height"=w1979:i32, "2 X"=w1980:i32, "1 Width"=w1981:i32, "In image?"=w1983:bool)  [unwired: 1 in]
                  n1273 = Not(x=w1983) -> (.not. x?=w1982:bool)
                }
              }
            }
            n1274 = Not(x=w1936) -> (.not. x?=w1935:bool)
            n1275 = case shown="True" w1935 {
              tunnel: w1933 -> [_ w1999]
              tunnel: w1931 -> [_ w1998]
              tunnel: w1934 -> [_ w1997]
              tunnel: w1932 -> [_ w1996]
              frame False {
              }
              frame True {
                w1992 = FALSE ("Get Point")
                n1276 = local read "Scan lines (y)"() -> (w2001:u64)
                n1277 = local read "Actual MCL Inc (V)"() -> (w1993:dbl)
                n1278 = local read "Scan steps (MCL)"() -> (w2000:u64)
                n1279 = Divide "Y Pix/step"(x=w1996, y=w2001) -> (x/y=w2008:dbl)
                n1280 = Divide "Y V/pix"(x=w1993, y=w2008) -> (x/y=w2007:dbl)
                n1281 = Divide "Y half step offset"(x=w1993, y=2.0) -> (x/y=w2009:dbl)
                n1282 = Divide "X pix/step"(x=w1997, y=w2000) -> (x/y=w2006:dbl)
                n1283 = Negate(x=w2009) -> (-x=w2010:dbl)
                n1284 = local read "Initial Y"() -> (w2016:dbl)
                n1285 = Multiply(x=w1998, y=w2007) -> (x*y=w2017:dbl)
                n1286 = Divide "X half step offset"(x=w1993, y=2.0) -> (x/y=w2003:dbl)
                n1287 = Divide "X V/pix"(x=w1993, y=w2006) -> (x/y=w2005:dbl)
                n1288 = Multiply(x=w1993, y=w2000) -> (x*y=w2012:dbl)
                n1289 = Compound Arithmetic op=ADD(w2010, w2017, w2016) -> (w1994:dbl)
                "Pointer Y (V)" <- w1994
                n1290 = Multiply(x=w2005, y=w1999) -> (x*y=w2014:dbl)
                n1291 = Negate(x=w2003) -> (-x=w2002:dbl)
                n1292 = local read "Initial X"() -> (w2015:dbl)
                n1293 = Negate(x=w2014) -> (-x=w2013:dbl)
                n1294 = Compound Arithmetic op=ADD(w2002, w2012, w2015, w2013) -> (w1995:dbl)
                "Pointer X (V)" <- w1995
                n1295 = Or(x="Set X Only", y="Set Confocal Spot (X-Y)") -> (x .or. y?=w1988:bool)
                n1296 = Or(x="Set Confocal Spot (X-Y)", y="Set Y Only") -> (x .or. y?=w1987:bool)
                n1297 = case shown="True" w1988 {
                  tunnel: w1995 -> [_ w2018]
                  frame False {
                  }
                  frame True {
                    n1298 = property on="AO2" class="Slide (strict)"("Val(Sgnl)"=w2018) -> ()  [unwired: 2 in, 2 out]
                  }
                }
                n1299 = case shown="True" w1987 {
                  tunnel: w1994 -> [_ w2019]
                  frame False {
                  }
                  frame True {
                    n1300 = property on="AO1" class="Slide (strict)"("Val(Sgnl)"=w2019) -> ()  [unwired: 2 in, 2 out]
                  }
                }
                n1301 = local write "Set Confocal Spot (X-Y)"(w1992) -> ()
                n1302 = local write "Set X Only"(w1992) -> ()
                n1303 = local write "Set Y Only"(w1992) -> ()
              }
            }
          }
          frame 3 {
            n1304 = local read "BD 2 Frequency 1 (MHz)"() -> (w2020:dbl)
            n1305 = local read "BD 1 Frequency 1 (MHz)"() -> (w2021:dbl)
            n1306 = local write "Manipulating Trap"(TRUE ("Manipulating Trap")) -> ()
            n1307 = local write "Coords"(T8 {"Horizontal"=0, "Vertical"=0} ("Coords")) -> ()
            n1308 = while {
              tunnel: w2026 -> [w2031]
              tunnel: w2024 -> [w2030]
              tunnel: w2022 -> [w2029]
              tunnel: w2021 -> [w2028]
              tunnel: w2020 -> [w2027]
              stop <- w2032 stop-if-true
              n1309 = event shown="[0] \"Pane\": Mouse Move" {
                selector: _ -> [_ _]
                dyn-events: _ -> [_ _]
                timeout: _ -> [_ _]
                tunnel: ["Force Manip Abort" w2096] -> w2032
                tunnel: w2031 -> [w2039 _]
                tunnel: w2030 -> [w2037 _]
                tunnel: w2029 -> [w2036 _]
                tunnel: w2028 -> [w2035 _]
                tunnel: w2027 -> [w2034 _]
                event Mouse Move {
                  n1310 = event-data() -> ("Time"=w2040:u32, "Coords"=w2041:T8)  [unwired: 3 out]
                  n1311 = Less?(x=w2040, y=w2039) -> (x < y?=w2038:bool)
                  n1312 = case "Makes sure old motion events prior to mouse click aren't used" shown="False" w2038 {
                    tunnel: w2041 -> [w2083 _]
                    tunnel: w2037 -> [w2084 _]
                    tunnel: w2036 -> [w2061 _]
                    tunnel: w2035 -> [w2057 _]
                    tunnel: w2034 -> [w2056 _]
                    frame False {
                      n1313 = Subtract(x=w2083, y=w2084) -> (x-y=w2082:T8)
                      "Coords" <- w2082
                      n1314 = local read "Y RF Frequency Limits (MHz)"() -> (w2042:T17)
                      n1315 = To Double Precision Float(number=w2082) -> (double precision float=w2081:cluster{"Horizontal":dbl, "Vertical":dbl})
                      n1316 = Multiply(x=cluster{"Horizontal":dbl, "Vertical":dbl} {"Horizontal"=-1.0, "Vertical"=1.0}, y="Manipulation Scaling") -> (x*y=w2077:cluster{"Horizontal":dbl, "Vertical":dbl})
                      n1317 = local read "X RF Frequency Limits (MHz)"() -> (w2043:T17)
                      n1318 = Multiply(x=w2081, y=w2077) -> (x*y=w2079:cluster{"Horizontal":dbl, "Vertical":dbl})
                      n1319 = Unbundle By Name(w2079) -> ("Horizontal"=w2074:dbl, "Vertical"=w2078:dbl)
                      n1320 = Unbundle By Name(w2042) -> ("Maximum"=w2045:dbl, "Minimum"=w2044:dbl)
                      n1321 = Boolean To (0,1)(Boolean="Manip. X?") -> (0, 1=w2072:i16)
                      n1322 = Boolean To (0,1)(Boolean="Manip. Y?") -> (0, 1=w2069:i16)
                      n1323 = local read "BD 1 Frequency 2 (MHz)"() -> (w2059:dbl)
                      n1324 = Multiply(x=w2078, y=w2069) -> (x*y=w2071:dbl)
                      n1325 = Multiply(x=w2072, y=w2074) -> (x*y=w2075:dbl)
                      n1326 = local read "BD 2 Frequency 2 (MHz)"() -> (w2058:dbl)
                      n1327 = Unbundle By Name(w2043) -> ("Maximum"=w2047:dbl, "Minimum"=w2046:dbl)
                      n1328 = Add(x=w2056, y=w2071) -> (x+y=w2049:dbl)
                      n1329 = Add(x=w2057, y=w2075) -> (x+y=w2051:dbl)
                      n1330 = In Range and Coerce(upper limit=w2047, x=w2051, lower limit=w2046) -> (coerced(x)=w2050:dbl)  [unwired: 1 out]
                      n1331 = In Range and Coerce(upper limit=w2045, x=w2049, lower limit=w2044) -> (coerced(x)=w2048:dbl)  [unwired: 1 out]
                      n1332 = Subtract(x=w2050, y=w2059) -> (x-y=w2068:dbl)
                      n1333 = Subtract(x=w2048, y=w2058) -> (x-y=w2067:dbl)
                      n1334 = Square(x=w2068) -> (x^2=w2066:dbl)
                      n1335 = Square(x=w2067) -> (x^2=w2065:dbl)
                      n1336 = Add(x=w2066, y=w2065) -> (x+y=w2064:dbl)
                      n1337 = Square Root(x=w2064) -> (sqrt(x)=w2060:dbl)
                      n1338 = In Range and Coerce(upper limit="Limit Max (MHz)", x=w2060, lower limit="Limit Min (MHz)") -> (In Range?=w2053:bool)  [unwired: 1 out]
                      n1339 = Not(x="Limits Enable") -> (.not. x?=w2052:bool)
                      n1340 = Or(x=w2053, y=w2052) -> (x .or. y?=w2054:bool)
                      n1341 = case shown="True" w2054 {
                        tunnel: w2061 -> [_ w2094]
                        tunnel: w2060 -> [_ w2085]
                        tunnel: w2050 -> [_ w2092]
                        tunnel: w2059 -> [_ w2091]
                        tunnel: w2048 -> [_ w2090]
                        tunnel: w2058 -> [_ w2089]
                        tunnel: w2043 -> [_ w2087]
                        tunnel: w2042 -> [_ w2086]
                        frame False {
                        }
                        frame True {
                          n1342 = local read "BD 1 Frequency 3 (MHz)"() -> (w2093:dbl)
                          n1343 = local read "BD 2 Frequency 3 (MHz)"() -> (w2088:dbl)
                          n1344 = local write "Trap Delta (MHz)"(w2085) -> ()
                          n1345 = property on="Initial delta (MHz)" class="DigNum (strict)"("Val(Sgnl)"=w2085) -> ()  [unwired: 2 in, 2 out]
                          n1346 = call "set RF board frequency - interlace.vi"("Board 2 Frequency Limits"=w2086, "Board 1 Frequency Limits"=w2087, "FPGA VI Reference In"=w2094, "Board 2 Frequency 3 (MHz)"=w2088, "Board 1 Frequency 3 (MHz)"=w2093, "Board 2 Frequency 2 (MHz)"=w2089, "Board 2 Frequency 1 (MHz)"=w2090, "Board 1 Frequency 2 (MHz)"=w2091, "Board 1 Frequency 1  (MHz)"=w2092) -> ()  [unwired: 1 in, 2 out]
                          n1347 = local write "BD 2 Frequency 1 (MHz)"(w2090) -> ()
                          n1348 = local write "BD 1 Frequency 1 (MHz)"(w2092) -> ()
                        }
                      }
                    }
                    frame True {
                    }
                  }
                }
                event Mouse Up {
                  n1349 = event-data() -> ("Button"=w2095:u16)  [unwired: 8 out]
